vi "SubscriberExample.vi"() -> ()   [LabVIEW 2012]
doc: "Sample subscriber that reads in a string from the publisher on the topic /chatter"
uses:
  <userlib>/ROS for LabVIEW Software/ROS/Code/Console/Servers/ServerSubs/TopicDef.ctl
  <userlib>/ROS for LabVIEW Software/ROS/Code/SubVIs/_ROSDirection.ctl
  <userlib>/ROS for LabVIEW Software/ROS/MessageParsing/std_msgs/subs/parse_string_scalar.vi
panel:
  in  "stop":bool
  out "error out":errorcluster
  out "I heard:":string
  # "Instructions:\n1. Run Publisher example\n2. Run Subscriber eample"
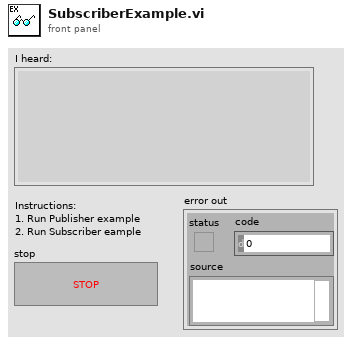
[diagram p1: front panel]
types:
  T1 = typedef "TopicDef.ctl" = cluster{"Topic":string, "Type":string, "Action":T2, "Update (ms)":u16, "queue size":u16}
  T2 = typedef "_ROSDirection.ctl" = enum16{"Node", "Publisher", "Subscriber", "ServiceClient", "ServiceProvider"}
  T3 = typedef "_ROSControl.ctl" = cluster{"topic port":u16, "Node":string, "topic":string, "type":string, "node port":u16, "error ":errorcluster, "Direction":T2, "Update (ms)":u16, "FIFO size":u16}
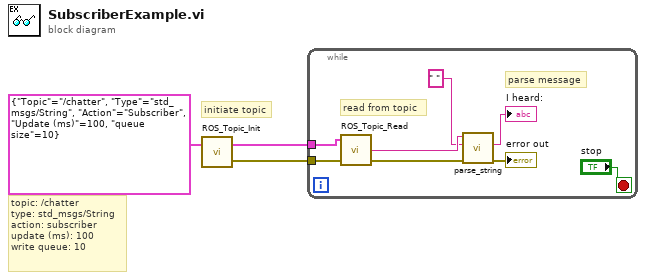
[diagram p0: block diagram]
diagram:
  # "initiate topic"
  # "topic: /chatter\ntype: std_msgs/String\naction: subscriber\nupdate (ms): 100\nwrite queue: 10"
  n1 = call <userlib>:"ROS_Topic_Init.vi"("Definitions"=T1 {"Topic"="/chatter", "Type"="std_msgs/String", "Action"=enum."Subscriber", "Update (ms)"=100, "queue size"=10}) -> ("error out"=w1:errorcluster, "ROS out"=w2:T3)  [unwired: 1 in]
  n2 = while {
    tunnel: w2 -> [w11]
    tunnel: w1 -> [w7]
    stop <- "stop" stop-if-true
    # "parse message"
    # "read from topic"
    n3 = call <userlib>:"ROS_Topic_Read.vi"("error in (no error)"=w7, "ROS in"=w11) -> ("error out"=w6:errorcluster, "Reply"=w10:string)  [unwired: 1 in, 1 out]
    n4 = call-poly <userlib>:"parse_string.vi"("error in"=w6, "type"=" ", "msg in"=w10) -> ("error out"=→"error out":errorcluster, "string"=→"I heard:":string)  [unwired: 2 in, 1 out]
  }
